vi "Cryo-Con Set H.vi"(8 "error in (no error)":errorcluster, 10 "Set T":T1=enum."0.25W", 11 "VISA Resource Name":refnum<visa-resource-name>) -> (0 "error out":errorcluster, 3 "VISA Resource Name Out":refnum<visa-resource-name>)   [LabVIEW 2015]
uses:
  Cryo-con Heater Ranges.ctl
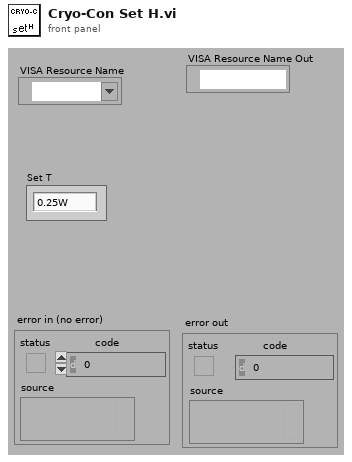
[diagram p1: front panel]
types:
  T1 = typedef "Cryo-con Heater Ranges.ctl" = enum16{"25W", "2.5W", "0.25W"}
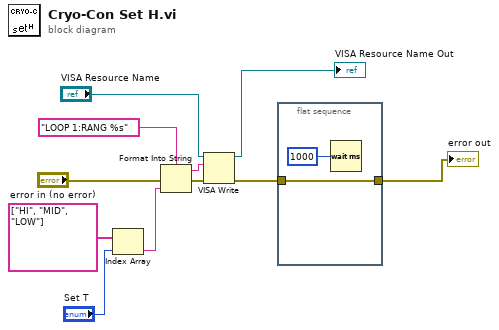
[diagram p0: block diagram]
diagram:
  n1 = Index Array(array=string[] ["HI", "MID", "LOW"] ("string array"), index="Set T") -> (element=w3:string)
  n2 = Format Into String(format string="LOOP 1:RANG %s", error in="error in (no error)", w3) -> (resulting string=w8:string, error out=w10:errorcluster)  [unwired: 1 in]
  n3 = VISA Write(VISA resource name="VISA Resource Name", write buffer=w8, error in (no error)=w10) -> (VISA resource name out=→"VISA Resource Name Out":refnum<visa-resource-name>, error out=w2:errorcluster)  [unwired: 1 out]
  n4 = flat-sequence {
    tunnel: w2 -> [w12]
    tunnel: [w12] -> w1
    frame #0 {
      n5 = Wait (ms)(milliseconds to wait=u32 1000) -> ()  [unwired: 1 out]
    }
  }
  "error out" <- w1
